vi "PopupDialog.vi"() -> ()   [LabVIEW 2018]
uses:
  Global 1.vi
panel:
  out "Alarm Display":string
  in  "Boolean":bool
  in  "Color":u32(colorbox)=16711680
  in  "Text":string
  out "String":string
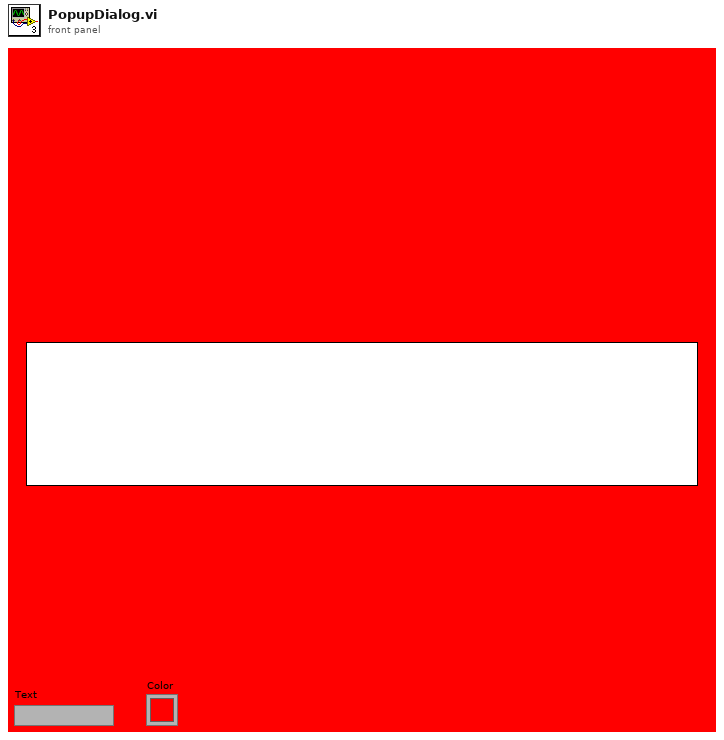
[diagram p1: front panel]
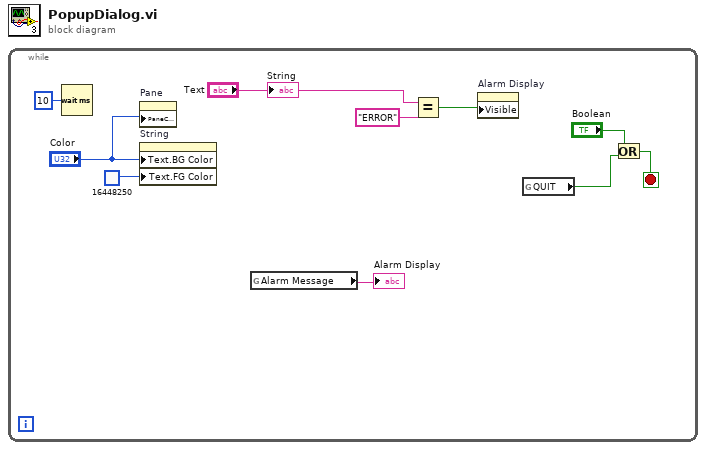
[diagram p0: block diagram]
diagram:
  n1 = while {
    stop <- w6 stop-if-true
    n2 = Wait (ms)(milliseconds to wait=u32 10) -> ()  [unwired: 1 out]
    n3 = property on="Pane" class="Pane"("PaneColor"="Color") -> ()  [unwired: 2 in, 2 out]
    n4 = property on="String" class="Str"("Text.BG Color"="Color", "Text.FG Color"=u32 16448250) -> ()  [unwired: 2 in, 2 out]
    n5 = global read "Global 1.vi" "Alarm Message"() -> (→"Alarm Display":string)
    n6 = Equal?(x="Text", y="ERROR") -> (x = y?=w3:bool)
    n7 = property on="Alarm Display" class="Str"("Visible"=w3) -> ()  [unwired: 2 in, 2 out]
    n8 = global read "Global 1.vi" "QUIT"() -> (w1:bool)
    n9 = Or(x="Boolean", y=w1) -> (x .or. y?=w6:bool)
    "String" <- "Text"
  }
